vi "set_config_cluster.vi"(8 "error in (no error)":errorcluster, 10 "config cluster variant":variant, 11 "DetectorDL090603DAQmxOnOff in":refnum<class "DetectorDL090603DAQmxOnOff.lvclass">) -> (0 "error out":errorcluster, 3 "DetectorDL090603DAQmxOnOff out":refnum<class "DetectorDL090603DAQmxOnOff.lvclass">)   [LabVIEW 2010, in "DetectorDL090603DAQmxOnOff.lvclass"]
uses:
  DetectorDL090603DAQmxOnOff.lvclass
  DetectorDL090603DAQmxOnOff.lvclass/DetectorDL090603DAQmxOnOff.ctl
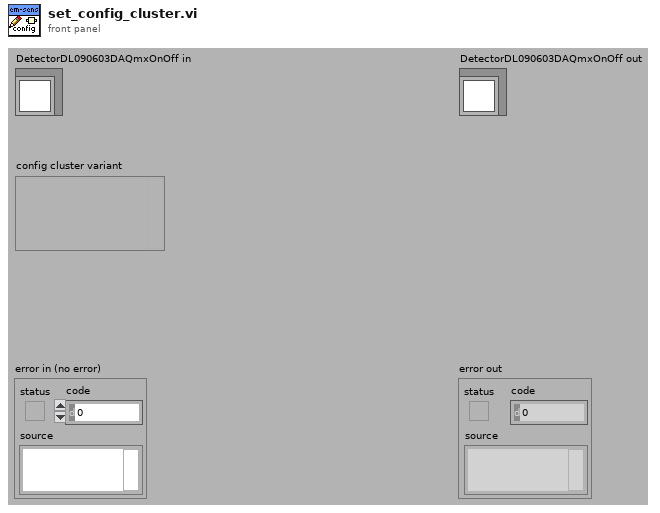
[diagram p1: front panel]
types:
  T1 = typedef "DetectorDL090603DAQmxOnOff.lvclass/config_data_cluster.ctl" = cluster{"DAQmxDigitalOut":T2, "specify voltage?":bool}
  T2 = typedef "plugin_specification.ctl" = cluster{"class path":string, "configuration":string, "label":string, "settings name":string}
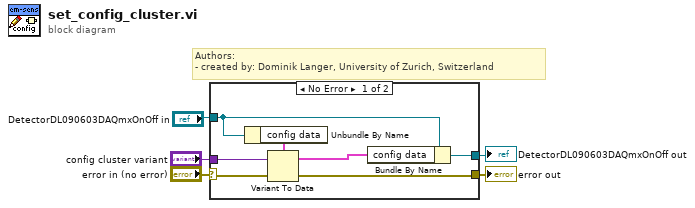
[diagram p0: block diagram]
diagram:
  # "Authors: \n- created by: Dominik Langer, University of Zurich, Switzerland"
  n1 = case shown="No Error" "error in (no error)" {
    selector: "error in (no error)" -> [w10 w13]
    tunnel: "config cluster variant" -> [w9 _]
    tunnel: "DetectorDL090603DAQmxOnOff in" -> [w8 w14]
    tunnel: [w6 w14] -> w2
    tunnel: [w7 w13] -> w1
    frame No Error {
      n2 = Unbundle By Name(w8) -> ("config data"=w11:T1)
      n3 = Variant To Data(error in=w10, Variant=w9, type=w11) -> (error out=w7:errorcluster, data=w12:T1)
      n4 = Bundle By Name(cluster=w8, "config data"=w12) -> (w6:refnum<class "DetectorDL090603DAQmxOnOff.lvclass">)
    }
    frame Error {
    }
  }
  "error out" <- w1
  "DetectorDL090603DAQmxOnOff out" <- w2
